vi "Get Value by Array (JSON).vi"(8 "error in (no error)":errorcluster, 10 "Keys":string[](array[string]), 11 "JSON Object in":refnum<class "JSON Object.lvclass">) -> (0 "error out":errorcluster, 2 "JSON Datatype out":refnum<class "JSON Null.lvclass">)   [LabVIEW 2015, in "LVJSON.lvlib" / "JSON Object.lvclass"]
uses:
  JSON Object.lvclass
  JSON Datatype/JSON Null.lvclass
  Errors/Errors.ctl
  JSON Helper/To More Specific Type (Object).vi
  Get Value (JSON).vi
  JSON Helper/To More Specific Type (Array).vi
  JSON Array/Index Array (JSON).vi
  JSON Helper/JSON Helper.lvclass
  JSON Array/JSON Array.lvclass
  LVJSON.lvlib
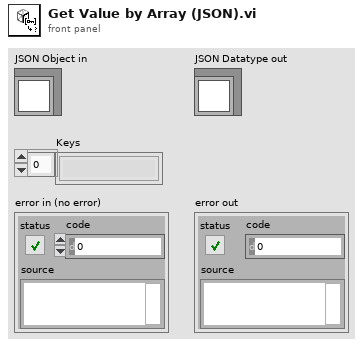
[diagram p1: front panel]
types:
  T1 = typedef "LVJSON.lvlib/Errors.ctl" = enum16{"No key", "Key path type", "Array OOB", "Type Mismatch", "Invalid Token"}
  T2 = typedef "LVJSON.lvlib/JSON Types.ctl" = enum16{"String", "Numeric", "Boolean", "NULL", "Object", "Array"}
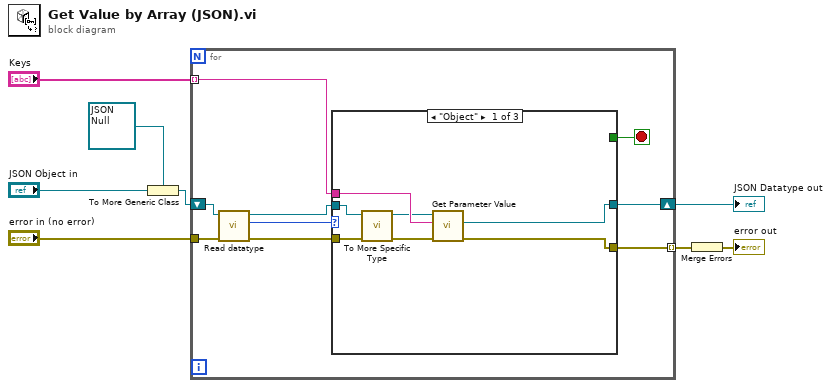
[diagram p0: block diagram]
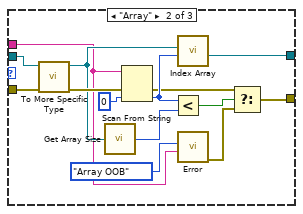
[diagram p2: hidden frame]
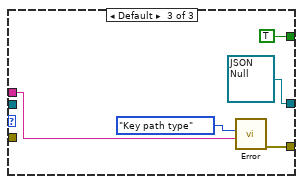
[diagram p3: hidden frame]
diagram:
  n1 = To More Generic Class(target class=refnum<class "JSON Null.lvclass"> refnum, reference="JSON Object in") -> (generic class reference=w5:refnum<class "JSON Null.lvclass">)
  n2 = for {
    tunnel: "Keys" -> [w17] mode=indexing
    shift-right: [w16] -> w7
    shift-left: w5 -> [w15]
    tunnel: "error in (no error)" -> [w13]
    tunnel: [w12] -> w2 mode=indexing
    stop <- w10 stop-if-true
    n3 = call-dynamic "Read datatype.vi"("error in (no error)"=w13, "JSON Datatype in"=w15) -> ("error out"=w11:errorcluster, "datatype"=w14:T2, "JSON Datatype out"=w9:refnum<class "JSON Null.lvclass">)  [unwired: 7 in]
    n4 = case shown="\"Object\"" w14 {
      tunnel: w17 -> [w24 w25 w39]
      tunnel: [w23 w36 refnum<class "JSON Null.lvclass"> refnum ("JSON Data")] -> w16
      tunnel: w9 -> [w21 w38 _]
      tunnel: [w18 w30 w41] -> w12
      tunnel: w11 -> [w20 w35 _]
      tunnel: [_ _ TRUE] -> w10
      frame "Object" {
        n5 = call-poly "To More Specific Type.vi"("error in (no error)"=w20, "JSON Datatype in"=w21) -> ("error out"=w19:errorcluster, "JSON Datatype out"=w22:refnum<class "JSON Object.lvclass">)  [unwired: 8 in]
        n6 = call-poly "Get Parameter Value.vi"("error in (no error)"=w19, "key"=w24, "JSON Object in"=w22) -> ("error out"=w18:errorcluster, "value"=w23:refnum<class "JSON Null.lvclass">)  [unwired: 7 in]
      }
      frame "Array" {
        n7 = call-poly "To More Specific Type.vi"("error in (no error)"=w35, "JSON Datatype in"=w38) -> ("error out"=w34:errorcluster, "JSON Datatype out"=w33:refnum<class "JSON Array.lvclass">)  [unwired: 8 in]
        n8 = call "Get Array Size.vi"("JSON Array in"=w33) -> ("size(s)"=w32:i32)
        n9 = Scan From String(input string=w25, error in=w34, default 1=0 ("index")) -> (error out=w28:errorcluster, output 1=w31:i32)  [unwired: 2 in, 2 out]
        n10 = Less?(x=w31, y=w32) -> (x < y?=w29:bool)
        n11 = call-poly "Index Array.vi"("index"=w31, "JSON Array in"=w33) -> ("JSON Data"=w36:refnum<class "JSON Null.lvclass">)  [unwired: 9 in]
        n12 = call "Error.vi"("Data"=w25, 9:Errors."Array OOB") -> ("error out"=w27:errorcluster)  [unwired: 8 in]
        n13 = Select(t=w28, s=w29, f=w27) -> (s? t:f=w30:errorcluster)
      }
      frame Default {
        n14 = call "Error.vi"("Data"=w39, 9:Errors."Key path type") -> ("error out"=w41:errorcluster)  [unwired: 8 in]
      }
    }
  }
  "JSON Datatype out" <- w7
  n15 = Merge Errors(w2) -> (→"error out":errorcluster)
